vi "FlatToRichrfcontrol_GetGPSUTCStartTimeRequest.vi"(5 "OutputClusterType":T1, 11 "InputCluster":T2) -> (3 "OutputCluster":T1)   [LabVIEW 2024, in "FlexSDR_gRPC_client.lvlib"]
uses:
  rfcontrol_GetGPSUTCStartTimeRequest_Flat.ctl
  rfcontrol_GetGPSUTCStartTimeRequest.ctl
  FlexSDR_gRPC_client.lvlib
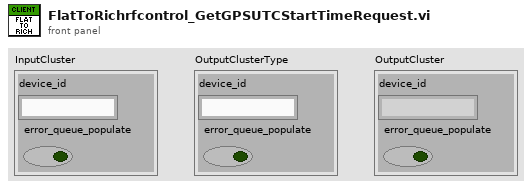
[diagram p1: front panel]
types:
  T1 = typedef "FlexSDR_gRPC_client.lvlib/rfcontrol_GetGPSUTCStartTimeRequest.ctl" = cluster{"device_id":string, "error_queue_populate":bool}
  T2 = typedef "FlexSDR_gRPC_client.lvlib/rfcontrol_GetGPSUTCStartTimeRequest_Flat.ctl" = cluster{"device_id":string, "error_queue_populate":bool}
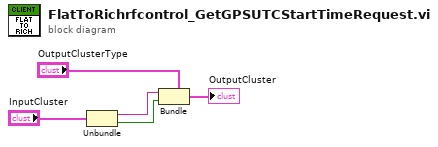
[diagram p0: block diagram]
diagram:
  n1 = Unbundle "Unbundle"("InputCluster") -> ("device_id"=w2:string, "error_queue_populate"=w1:bool)
  n2 = Bundle "Bundle"(cluster="OutputClusterType", "device_id"=w2, "error_queue_populate"=w1) -> (→"OutputCluster":T1)
